vi "通讯.vi"() -> ()   [LabVIEW 2016, in "流量计集成.lvlib" / "博意达流量计.lvlib"]
uses:
  <vilib>/Analysis/baseanly.llb/Mean (DBL).vi
  <vilib>/Plasmionique/MB Master/MB_Master_Serial/MB_Master_Serial.lvclass
  D:/Program Files (x86)/National Instruments/LabVIEW 2016/vi.lib/Plasmionique/MB Master/MB_Master/MB_Master.lvclass
  <vilib>/Analysis/NI_AALBase.lvlib
  <vilib>/Plasmionique/MB Master/MB Master.lvlib
panel:
  in  "停止":bool
  out "水温":dbl[](array[numeric])
  out "总累积流量":dbl
  out "总流量":dbl
  out "平均流速":dbl
  out "平均水位":dbl
  out "累积流量":dbl[](array[numeric])
  out "流速":dbl[](array[numeric])
  out "流量":dbl[](array[numeric])
  out "水位":dbl[](array[numeric])
  out "流量计启用":bool[](array[boolean])
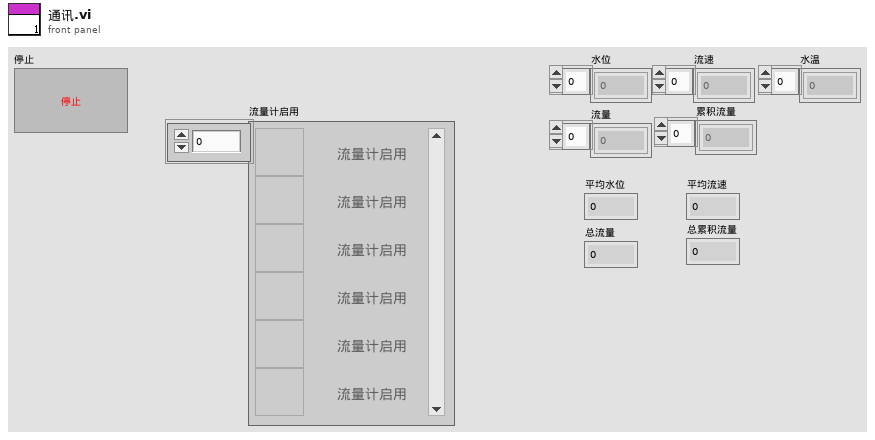
[diagram p1: front panel]
types:
  T1 = cluster{"baud rate (bps)":u32, "stop bits":u16, "parity":u16, "flow control":u16, "timeout":u32, "retries":i32}
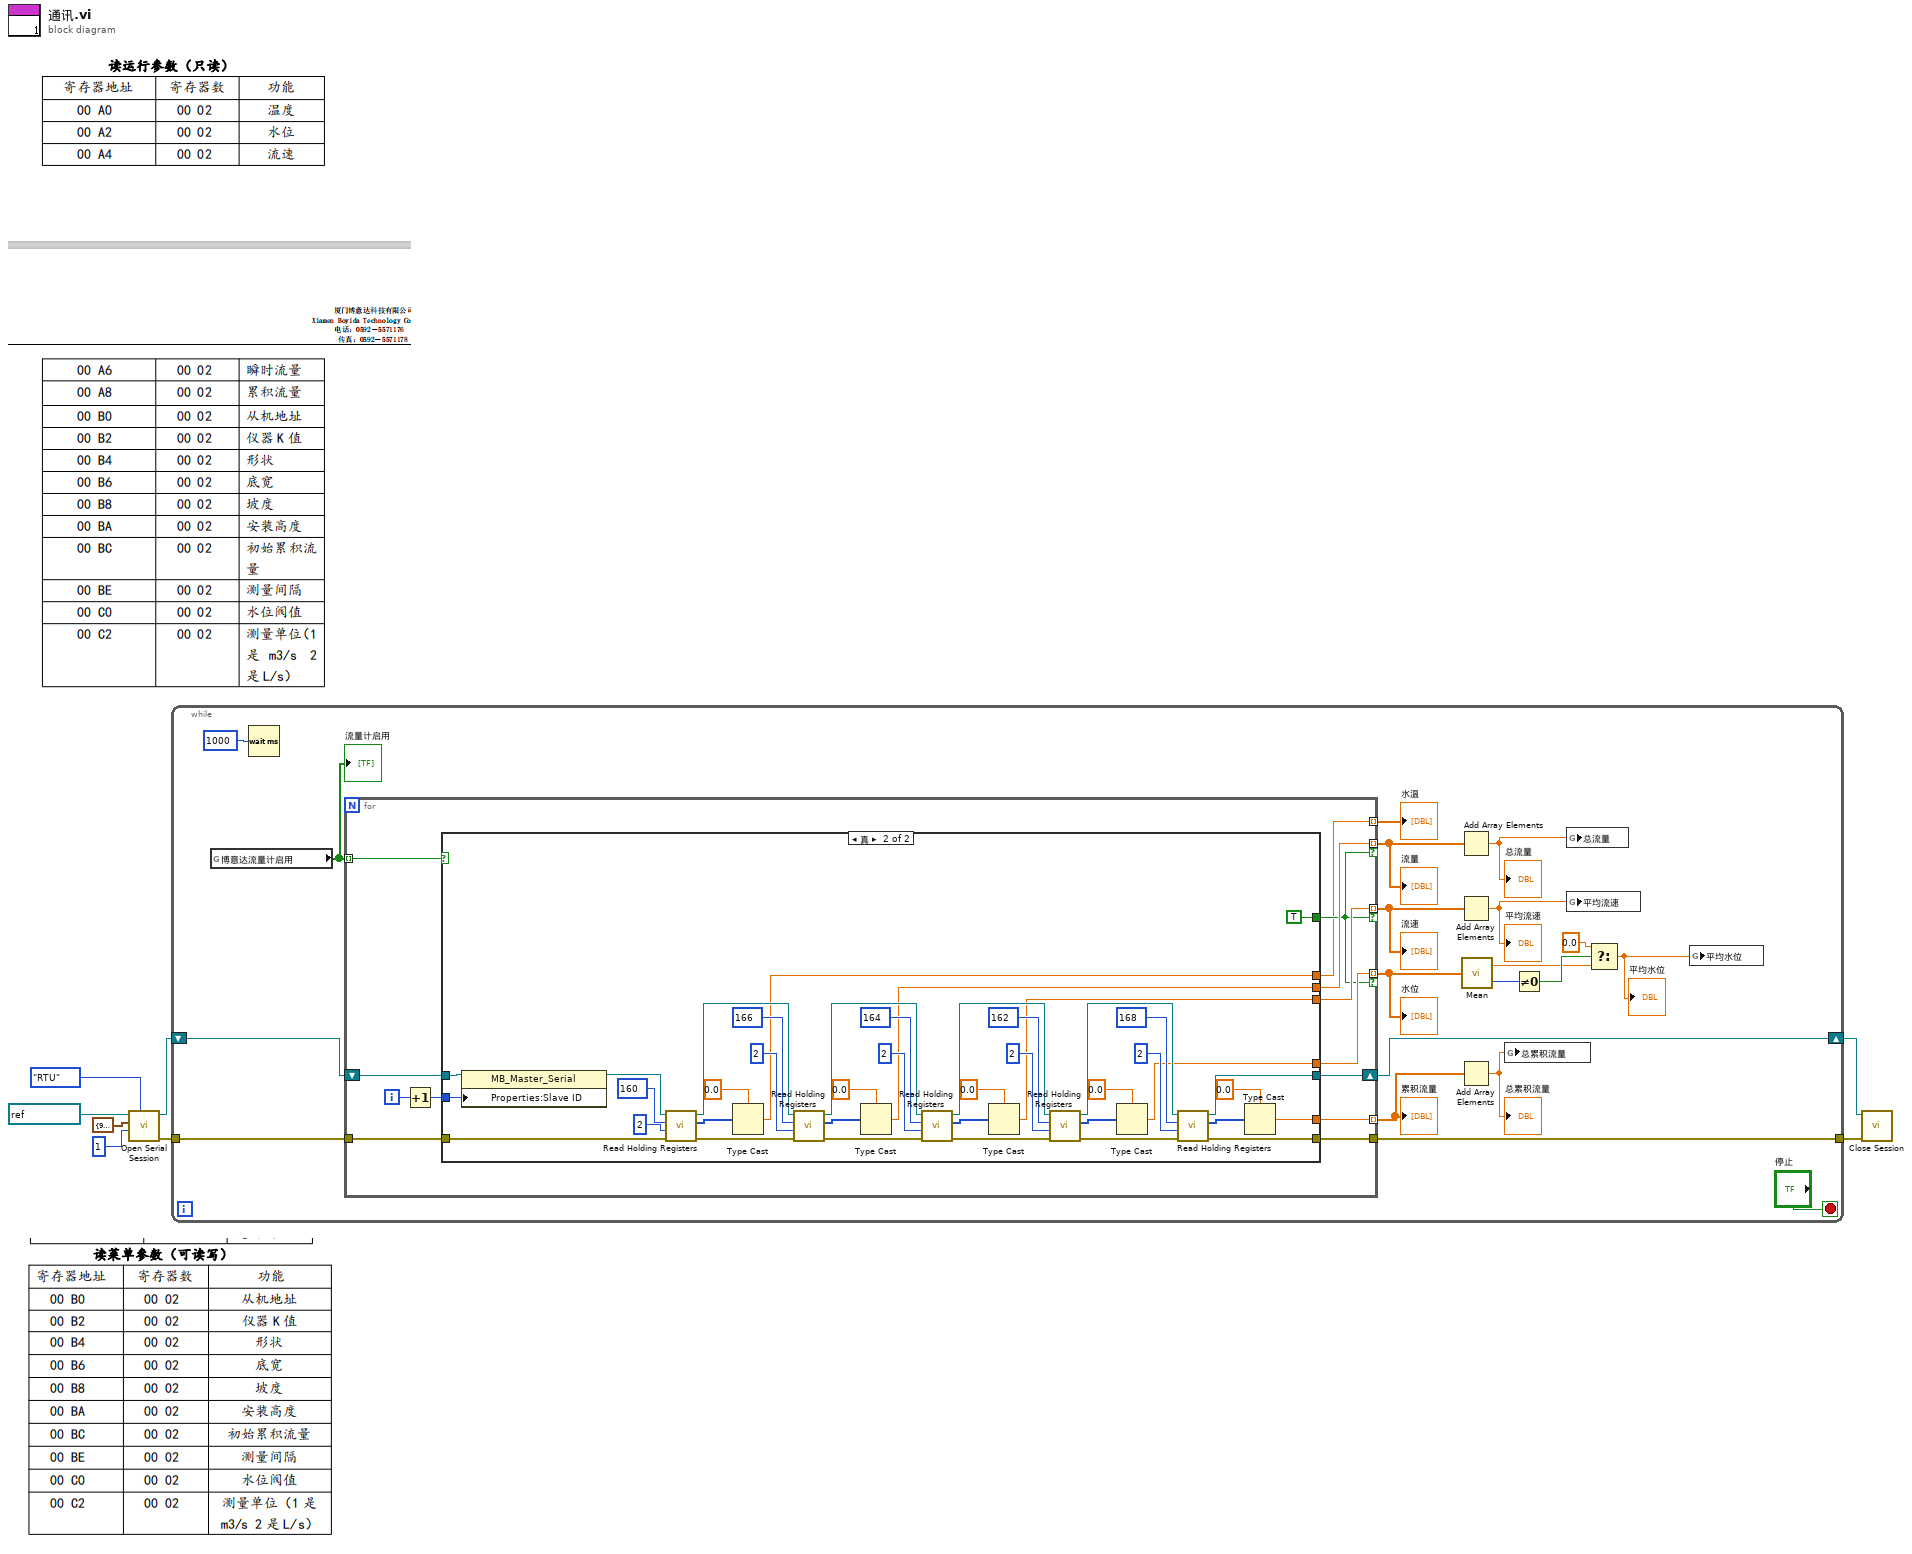
[diagram p0: block diagram]
diagram:
  n1 = call <vilib>:"Open Serial Session.vi"("Mode (RTU)"=enum16{"RTU", "ASCII"}."RTU", "Slave ID"=u8 1, "Serial Config"=T1 {"baud rate (bps)"=9600, "stop bits"=10, "parity"=0, "flow control"=0, "timeout"=1000, "retries"=1}, "VISA Resource"=refnum<visa-resource-name> "COM10") -> ("Error out"=w6:errorcluster, "MB_Serial session"=w1:refnum<class "MB_Master_Serial.lvclass">)  [unwired: 6 in]
  n2 = while {
    tunnel: w6 -> [w28]
    shift-right: [w27] -> w8
    shift-left: w1 -> [w24]
    tunnel: [w26] -> w7
    stop <- "停止" stop-if-true
    n3 = global read "流量计全局变量.vi" "博意达流量计启用"() -> (w12:bool[])
    "流量计启用" <- w12
    n4 = Wait (ms)(milliseconds to wait=u32 1000 ("等待时间（毫秒）")) -> ()  [unwired: 1 out]
    n5 = for {
      shift-right: [w40] -> w27
      shift-left: w24 -> [w38]
      tunnel: w12 -> [w35] mode=indexing
      tunnel: [w34] -> w22 mode=indexing if=w31
      tunnel: [w33] -> w23 mode=indexing if=w31
      tunnel: [w32] -> w19 mode=indexing if=w31
      tunnel: w28 -> [w41]
      tunnel: [w39] -> w26
      tunnel: [w30] -> w11 mode=indexing
      tunnel: [w29] -> w9 mode=indexing
      i -> [w37]
      n6 = Increment(x=w37) -> (x+1=w36:i32)
      n7 = case shown="真" w35 {
        tunnel: w41 -> [w42 w49]
        tunnel: [w43 w45] -> w40
        tunnel: [w42 w44] -> w39
        tunnel: w38 -> [w43 w83]
        tunnel: w36 -> [_ w82]
        tunnel: [_ w56] -> w34
        tunnel: [_ w55] -> w33
        tunnel: [_ w58] -> w29
        tunnel: [_ w57] -> w32
        tunnel: [_ TRUE] -> w31
        tunnel: [_ w46] -> w30
        frame False {
        }
        frame True {
          n8 = property class="MB_Master_Serial"(reference=w83, "Properties:Slave ID"=w82) -> (reference out=w50:refnum<class "MB_Master_Serial.lvclass">)  [unwired: 1 in, 1 out]
          n9 = call <vilib>:"Read Holding Registers.vi"("error in (no error)"=w49, "quantity"=u16 2, "starting address"=u16 160, "MB session in"=w50) -> ("error out"=w48:errorcluster, "Registers"=w52:u16[], "MB session out"=w47:refnum<class "MB_Master_Serial.lvclass">)  [unwired: 5 in]
          n10 = Type Cast(type=sgl 0.0 ("x/y"), x=w52) -> (*(type *) &x=w46:sgl)
          n11 = call <vilib>:"Read Holding Registers.vi"("error in (no error)"=w48, "quantity"=u16 2, "starting address"=u16 166, "MB session in"=w47) -> ("error out"=w78:errorcluster, "Registers"=w70:u16[], "MB session out"=w79:refnum<class "MB_Master_Serial.lvclass">)  [unwired: 5 in]
          n12 = Type Cast(type=sgl 0.0 ("x/y"), x=w70) -> (*(type *) &x=w56:sgl)
          n13 = call <vilib>:"Read Holding Registers.vi"("error in (no error)"=w78, "quantity"=u16 2, "starting address"=u16 164, "MB session in"=w79) -> ("error out"=w74:errorcluster, "Registers"=w69:u16[], "MB session out"=w76:refnum<class "MB_Master_Serial.lvclass">)  [unwired: 5 in]
          n14 = Type Cast(type=sgl 0.0 ("x/y"), x=w69) -> (*(type *) &x=w57:sgl)
          n15 = call <vilib>:"Read Holding Registers.vi"("error in (no error)"=w74, "quantity"=u16 2, "starting address"=u16 162, "MB session in"=w76) -> ("error out"=w72:errorcluster, "Registers"=w68:u16[], "MB session out"=w73:refnum<class "MB_Master_Serial.lvclass">)  [unwired: 5 in]
          n16 = Type Cast(type=sgl 0.0 ("x/y"), x=w68) -> (*(type *) &x=w55:sgl)
          n17 = call <vilib>:"Read Holding Registers.vi"("error in (no error)"=w72, "quantity"=u16 2, "starting address"=u16 168, "MB session in"=w73) -> ("error out"=w44:errorcluster, "Registers"=w62:u16[], "MB session out"=w45:refnum<class "MB_Master_Serial.lvclass">)  [unwired: 5 in]
          n18 = Type Cast(type=sgl 0.0 ("x/y"), x=w62) -> (*(type *) &x=w58:sgl)
        }
      }
    }
    "水位" <- w23
    "流量" <- w22
    "流速" <- w19
    "累积流量" <- w9
    "水温" <- w11
    n19 = Add Array Elements(numeric array=w22) -> (sum=w20:sgl)
    "总流量" <- w20
    n20 = Add Array Elements(numeric array=w19) -> (sum=w18:sgl)
    "平均流速" <- w18
    n21 = Add Array Elements(numeric array=w9) -> (sum=w21:sgl)
    "总累积流量" <- w21
    n22 = call-poly <vilib>:"Mean.vi"("X"=w23) -> ("mean"=w14:dbl, "error"=w17:i32)
    n23 = global write "流量计全局变量.vi" "总累积流量"(w21) -> ()
    n24 = Not Equal To 0?(x=w17) -> (x != 0?=w16:bool)
    n25 = global write "流量计全局变量.vi" "总流量"(w20) -> ()
    n26 = global write "流量计全局变量.vi" "平均流速"(w18) -> ()
    n27 = Select(t=0.0, s=w16, f=w14) -> (s? t:f=w13:dbl)
    "平均水位" <- w13
    n28 = global write "流量计全局变量.vi" "平均水位"(w13) -> ()
  }
  n29 = call-dynamic "Close Session.vi"("error in (no error)"=w7, "MB_Serial session"=w8) -> ()  [unwired: 9 in, 1 out]
